vi "Get Tx Channel Array.vi"() -> (1 "Channel Array":string[](array[string]))   [LabVIEW 2020, in "afdx_custom_device GUID Utility.lvlib"]
uses:
  Scripting/Constants.vi
  afdx_custom_device GUID Utility.lvlib
  Scripting/afdx_custom_device Scripting.lvlib
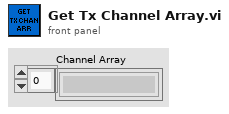
[diagram p1: front panel]
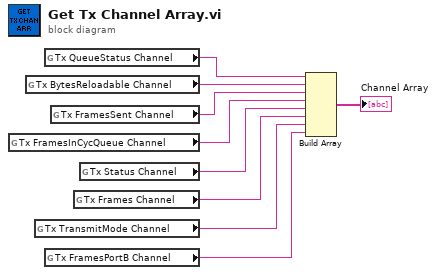
[diagram p0: block diagram]
diagram:
  n1 = global read "Constants.vi" "Tx FramesInCycQueue Channel"() -> (w7:string)
  n2 = global read "Constants.vi" "Tx BytesReloadable Channel"() -> (w9:string)
  n3 = global read "Constants.vi" "Tx TransmitMode Channel"() -> (w4:string)
  n4 = global read "Constants.vi" "Tx QueueStatus Channel"() -> (w1:string)
  n5 = global read "Constants.vi" "Tx FramesPortB Channel"() -> (w3:string)
  n6 = global read "Constants.vi" "Tx FramesSent Channel"() -> (w8:string)
  n7 = global read "Constants.vi" "Tx Frames Channel"() -> (w5:string)
  n8 = global read "Constants.vi" "Tx Status Channel"() -> (w6:string)
  n9 = Build Array(w1, w9, w8, w7, w6, w5, w4, w3) -> (→"Channel Array":string[])
